vi "calibrationElectrometer_getEvent_LargeFileObjectAvailable.vi"(8 "error in (no error)":errorcluster, 11 "logevent_LargeFileObjectAvailable_Ctl":T1={"URL"="", "Generator"="", "Version"=0.0, "Checksum"="", "Mime_Type"="                                ", "Byte_Size"=0, "ID"="", "priority"=0}) -> (0 "error out":errorcluster, 2 "function return":i32, 3 "logevent_LargeFileObjectAvailable_Ctl out":T1={"URL"="", "Generator"="", "Version"=0.0, "Checksum"="", "Mime_Type"="                                ", "Byte_Size"=0, "ID"="", "priority"=0})   [LabVIEW 2016, in "SALLV_calibrationElectrometer.lvlib"]
doc: "int calibrationElectrometer_shm_getEvent_LargeFileObjectAvailableLV(calibrationElectrometer_logevent_LargeFileObjectAvailableLV *logevent_LargeFileObjectAvailable_Ctl );"
uses:
  SALLV_calibrationElectrometer.lvlib
  DataTypes/logevent_LargeFileObjectAvailable.ctl
  SALLV_calibrationElectrometer.so
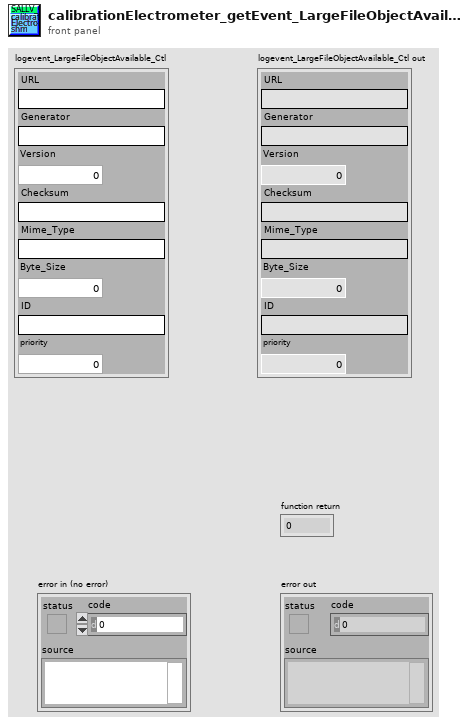
[diagram p1: front panel]
types:
  T1 = typedef "SALLV_calibrationElectrometer.lvlib/logevent_LargeFileObjectAvailable.ctl" = cluster{"URL":string, "Generator":string, "Version":sgl, "Checksum":string, "Mime_Type":string, "Byte_Size":i32, "ID":string, "priority":i32}
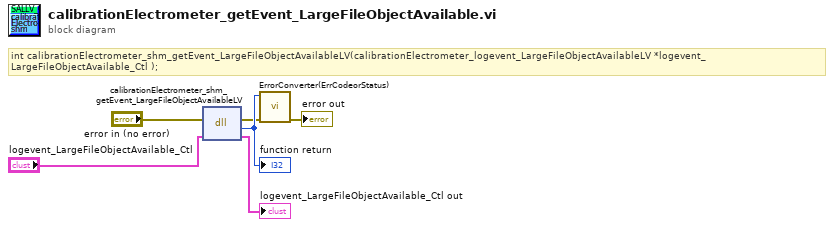
[diagram p0: block diagram]
diagram:
  # "int calibrationElectrometer_shm_getEvent_LargeFileObjectAvailableLV(calibrationElectrometer_logevent_LargeFileObjectAvailableLV *logevent_LargeFileObjectAvailable_Ctl );"
  n1 = dll-call lib="home/saluser/Desktop/SAL_Electrometer/SALLV_calibrationElectrometer.*" fn="calibrationElectrometer_shm_getEvent_LargeFileObjectAvailableLV"(error in="error in (no error)", "logevent_LargeFileObjectAvailable_Ctl"="logevent_LargeFileObjectAvailable_Ctl") -> (error out=w2:errorcluster, w6:i32, "logevent_LargeFileObjectAvailable_Ctl"=→"logevent_LargeFileObjectAvailable_Ctl out":T1)  [unwired: 2 in, 1 out]
  "function return" <- w6
  n2 = call "ErrorConverter(ErrCodeorStatus).vi"("error in (no error)"=w2, "error code"=w6) -> ("error out"=→"error out":errorcluster)  [unwired: 9 in]
